vi "Read Channels.vi"(8 "error in (no error)":errorcluster, 11 "Configuration.Transfer in":refnum<class "Configuration.Transfer.lvclass">) -> (0 "error out":errorcluster, 2 "Channels":refnum<class "Configuration.Channel.lvclass">[](array[class]), 3 "Configuration.Transfer out":refnum<class "Configuration.Transfer.lvclass">)   [LabVIEW 2016, in "Configuration.Transfer.lvclass"]
uses:
  Configuration.Transfer.lvclass
  Configuration.Channel/Configuration.Channel.lvclass
  Configuration.Transfer.lvclass/Configuration.Transfer.ctl
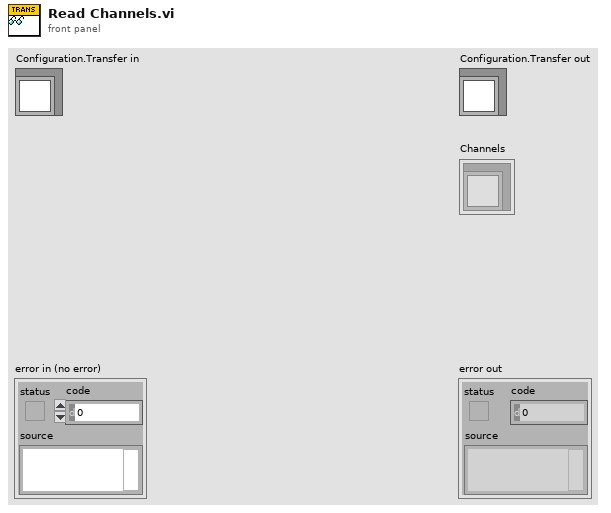
[diagram p1: front panel]
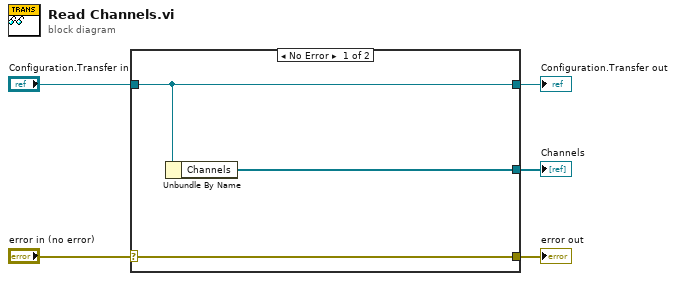
[diagram p0: block diagram]
diagram:
  n1 = case shown="No Error" "error in (no error)" {
    selector: "error in (no error)" -> [w8 w9]
    tunnel: [w8 w9] -> w4
    tunnel: [w7 w10] -> w2
    tunnel: "Configuration.Transfer in" -> [w7 w10]
    tunnel: [w6 _] -> w1
    frame No Error {
      n2 = Unbundle By Name(w7) -> ("Channels"=w6:refnum<class "Configuration.Channel.lvclass">[])
    }
    frame Error {
    }
  }
  "error out" <- w4
  "Configuration.Transfer out" <- w2
  "Channels" <- w1
